vi "Default UDP Delta.vi"() -> (3 "String":string)   [LabVIEW 2016]
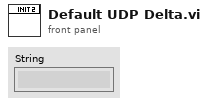
[diagram p1: front panel]
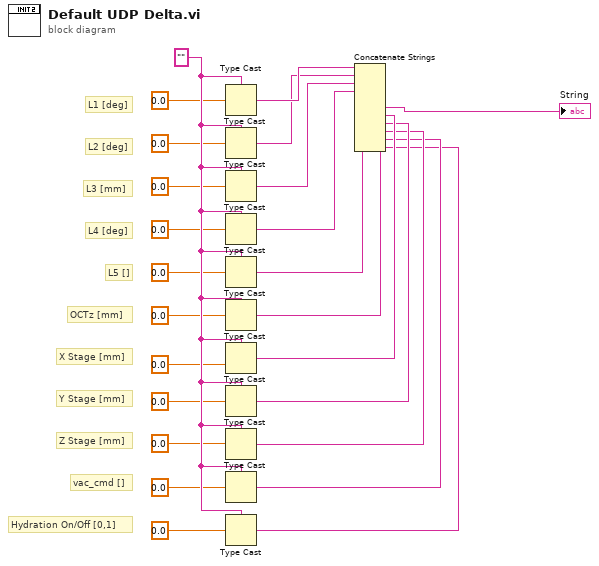
[diagram p0: block diagram]
diagram:
  w20 = "" ("data in")
  # "Hydration On/Off [0,1]"
  # "vac_cmd []"
  # "Z Stage [mm]"
  # "Y Stage [mm]"
  # "X Stage [mm]"
  # "OCTz [mm]"
  # "L5 []"
  # "L4 [deg]"
  # "L3 [mm]"
  # "L2 [deg]"
  # "L1 [deg]"
  n1 = Type Cast(type=w20, x=sgl 0.0 ("number")) -> (*(type *) &x=w23:string)
  n2 = Type Cast(type=w20, x=sgl 0.0 ("number")) -> (*(type *) &x=w21:string)
  n3 = Type Cast(type=w20, x=sgl 0.0 ("number")) -> (*(type *) &x=w22:string)
  n4 = Type Cast(type=w20, x=sgl 0.0 ("number")) -> (*(type *) &x=w19:string)
  n5 = Type Cast(type=w20, x=sgl 0.0 ("number")) -> (*(type *) &x=w18:string)
  n6 = Type Cast(type=w20, x=sgl 0.0 ("number")) -> (*(type *) &x=w17:string)
  n7 = Type Cast(type=w20, x=sgl 0.0 ("number")) -> (*(type *) &x=w16:string)
  n8 = Type Cast(type=w20, x=sgl 0.0 ("number")) -> (*(type *) &x=w15:string)
  n9 = Type Cast(type=w20, x=sgl 0.0 ("number")) -> (*(type *) &x=w14:string)
  n10 = Type Cast(type=w20, x=sgl 0.0 ("number")) -> (*(type *) &x=w13:string)
  n11 = Type Cast(type=w20, x=sgl 0.0 ("number")) -> (*(type *) &x=w12:string)
  n12 = Concatenate Strings(w23, w21, w22, w19, w18, w17, w16, w15, w14, w13, w12) -> (→"String":string)
